vi "AsyncEngine.CAN.vi"(10 "Parameters":variant, 11 "Process":refnum<class "Process.lvclass">) -> ()   [LabVIEW 2015, in "Protection and Rolling Counter Addon Engine.lvlib"]
uses:
  Protection and Rolling Counter Addon Engine.lvlib
  <vilib>/NI/NIVS Inline Async API/_VS Inline Async API/Process/Process.lvclass
  Types/RT Async Engine Variables.ctl
  Types/RT Frame Settings.ctl
  Types/RT Protection Configuration.ctl
  Shared/Types/Protection Type.ctl
  Shared/Types/InputChannelConfiguration.ctl
  Types/RT Counter Settings.ctl
  Types/RT Data References.ctl
  <vilib>/NI/NIVS Inline Async API/_Data Access Engine/Data Access Engine/Types/Write.DVR.ctl
  <vilib>/NI/NIVS Inline Async API/_Data Access Engine/Access Type Classes/Write/Write.lvclass
  <vilib>/NI/NIVS Inline Async API/_Data Access Engine/Data Access Engine/Types/Read.DVR.ctl
  <vilib>/NI/NIVS Inline Async API/_Data Access Engine/Access Type Classes/Read/Read.lvclass
  <vilib>/NI/NIVS Inline Async API/_VS Inline Async API/Process/Process.lvclass/Process.ctl
  <vilib>/Platform/TimedLoop/XDataNode/timing_clust.ctl
  <vilib>/Platform/TimedLoop/XDataNode/nitl_modes.ctl
  <vilib>/Platform/TimedLoop/XDataNode/wakeup.ctl
  <vilib>/NI/NIVS Inline Async API/_VS Inline Async API/Process/Data Member Access/Read Data Access.vi
  <vilib>/NI/NIVS Inline Async API/_VS Inline Async API/Error Handling Process/SubVIs/Error.ConvertArray.vi
  <vilib>/NI/NIVS Inline Async API/_Data Access Engine/Data Access Engine/Methods/Write.Lookup.vi
  <vilib>/NI/NIVS Inline Async API/_Data Access Engine/Data Access Engine/Methods/Read.Lookup.vi
  Shared/SubVIs/GUID Lookup.vi
  <vilib>/platform/TimedLoop/XDataNode/XDataNode.xnode
  <vilib>/NI/NIVS Inline Async API/_Data Access Engine/Data Access Engine/Data Access Engine.lvclass
  Shared/Protection and Rolling Counter Addon Shared.lvlib
  <vilib>/Platform/TimedLoop/XDataNode/XDNodeRunTimeDep.lvlib
  <vilib>/NI Veristand/Custom Device Tools/Custom Device Utility Library/Custom Device Utility Library.lvlib
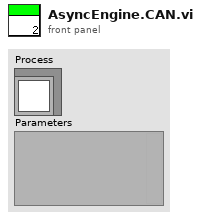
[diagram p1: front panel]
types:
  T1 = typedef "Protection and Rolling Counter Addon Engine.lvlib/RT Data References.ctl" = cluster{"ProtectionsAndCounters.Ref":T2, "Signals.Ref":T3, "Status.Ref":T2}
  T2 = typedef "Data Access Engine.lvlib/Data Access Engine.lvclass/Write.DVR.ctl" = refnum<data-value>
  T3 = typedef "Data Access Engine.lvlib/Data Access Engine.lvclass/Read.DVR.ctl" = refnum<data-value>
  T4 = typedef "Protection and Rolling Counter Addon Engine.lvlib/RT Async Engine Variables.ctl" = cluster{"CAN Session":refnum<k21>, "Frames":T5[], "Frame Count":i32}
  T5 = typedef "Protection and Rolling Counter Addon Engine.lvlib/RT Frame Settings.ctl" = cluster{"Frame ID":u32, "VS Offset":i32, "VS Length":i32, "Frame Conversion":refnum<k21>, "Generation Period":u32, "Time Since Last Generation":u32, "Has Protection?":bool, "Protection Configurations":T6[], "Has Counter":bool, "Counter Configurations":T9[], "Has Disable?":bool, "Disable VS Index":i32, "Frame.PrevData":dbl[], "Generation Iterations":u32, "Generation Counter":u32}
  T6 = typedef "Protection and Rolling Counter Addon Engine.lvlib/RT Protection Configuration.ctl" = cluster{"Protection Frame Index":i32, "Protection Type":T7, "Data Indeces":i32[], "Initialized Data Array":dbl[], "Check Sum Conversion":refnum<k21>, "CRC Channels":T8[], "Protection VS Index":i32}
  T7 = typedef "Protection and Rolling Counter Addon Shared.lvlib/Protection Type.ctl" = enum16{"Checksum", "CRC"}
  T8 = typedef "Protection and Rolling Counter Addon Shared.lvlib/InputChannelConfiguration.ctl" = cluster{"Start Bit":i32, "Name":string, "Number of bits":i32, "Scale":dbl, "Offset":dbl, "Data Type":u32}
  T9 = typedef "Protection and Rolling Counter Addon Engine.lvlib/RT Counter Settings.ctl" = cluster{"Counter Frame Index":i32, "Max Count":dbl, "Counter VS Index":i32}
  T10 = typedef "XDNodeRunTimeDep.lvlib/timing_clust.ctl" = cluster{"Expected End [f-1]":u64, "Actual End [f-1]":u64, "Finished Late? [f-1]":bool, "Expected End [i-1]":u64, "Actual End [i-1]":u64, "Finished Late? [i-1]":bool, "Expected Start [i]":u64, "Actual Start [i]":u64, "Expected Start [f]":u64, "Actual Start [f]":u64, "Source Name":string, "Structure Name":string, "Period":i64, "Deadline":i64, "Offset":i64, "Start":i64, "Priority":i32, "Timeout":i32, "Mode":T11, "Wakeup Reason":T12, "Error":errorcluster, "Source Type":string, "Secondary Source Type":string, "Global End Time":u64, "Global Start Time":u64, "Frame Duration":u64, "Iteration Duration":u64, "Assigned CPU":i32, "I/O Scan Engine Mode":u32}
  T11 = typedef "XDNodeRunTimeDep.lvlib/nitl_modes.ctl" = enum32{"No Change", "Process missed periods, maintain original phase", "Discard missed periods, maintain original phase", "Process missed periods, ignore original phase", "Discard missed periods, ignore original phase"}
  T12 = typedef "XDNodeRunTimeDep.lvlib/wakeup.ctl" = enum32{"Normal", "Aborted", "Asynchronous wakeup", "Timing source error", "Timed loop error", "Timeout"}
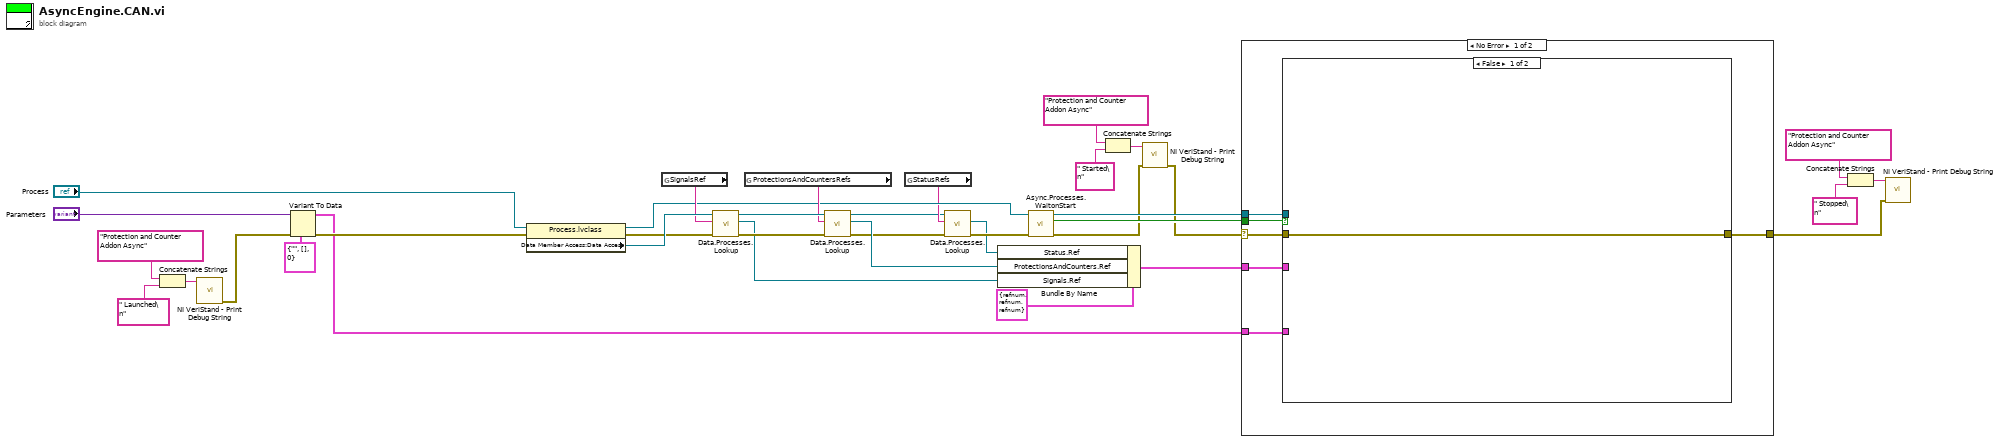
[diagram p0: block diagram]
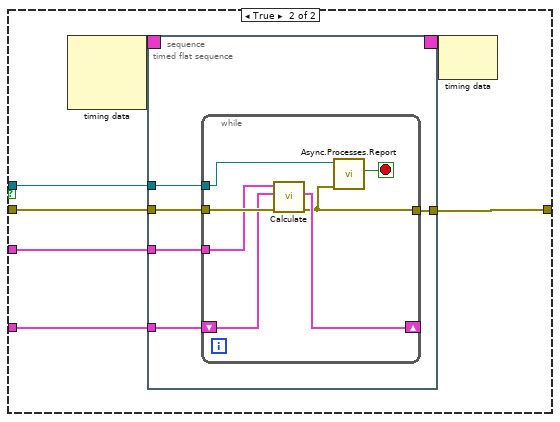
[diagram p2: hidden frame]
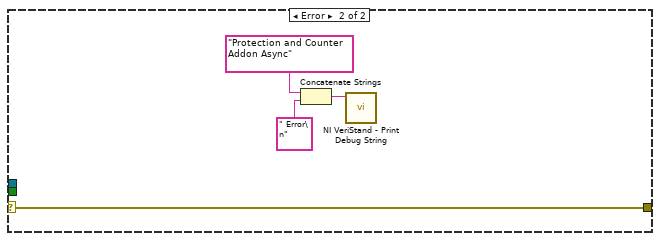
[diagram p3: hidden frame]
diagram:
  n1 = Concatenate Strings("Protection and Counter Addon Async" ("Debug String"), " Launched\n" ("string")) -> (w12:string)
  n2 = call <vilib>:"NI VeriStand - Print Debug String.vi"("Message"=w12) -> ("error out"=w10:errorcluster)  [unwired: 10 in]
  n3 = Variant To Data(error in=w10, type=T4 {"CAN Session"="", "Frames"=[], "Frame Count"=0} ("RT Configuration"), Variant="Parameters") -> (data=w20:T4, error out=w34:errorcluster)
  n4 = property class="Process.lvclass"(reference="Process", error in=w34) -> (reference out=w26:refnum<class "Process.lvclass">, error out=w30:errorcluster, "Data Member Access:Data Access"=w32:refnum<class "Data Access Engine.lvclass">)
  n5 = global read "GUID Lookup.vi" "SignalsRef"() -> (w28:string)
  n6 = call-poly <vilib>:"Data.Processes.Lookup.vi"("error in (no error)"=w30, "Name"=w28, "Data Access API in"=w32) -> ("error out"=w29:errorcluster, "Ref"=w24:T3, "Data Access API out"=w31:refnum<class "Data Access Engine.lvclass">)  [unwired: 5 in, 1 out]
  n7 = global read "GUID Lookup.vi" "ProtectionsAndCountersRefs"() -> (w27:string)
  n8 = call-poly <vilib>:"Data.Processes.Lookup.vi"("error in (no error)"=w29, "Name"=w27, "Data Access API in"=w31) -> ("error out"=w16:errorcluster, "Ref"=w23:T2, "Data Access API out"=w17:refnum<class "Data Access Engine.lvclass">)  [unwired: 5 in, 1 out]
  n9 = global read "GUID Lookup.vi" "StatusRefs"() -> (w18:string)
  n10 = call-poly <vilib>:"Data.Processes.Lookup.vi"("error in (no error)"=w16, "Name"=w18, "Data Access API in"=w17) -> ("error out"=w15:errorcluster, "Ref"=w14:T2)  [unwired: 5 in, 2 out]
  n11 = Bundle By Name(cluster=T1 {"ProtectionsAndCounters.Ref"=refnum, "Signals.Ref"=refnum, "Status.Ref"=refnum}, "Status.Ref"=w14, "ProtectionsAndCounters.Ref"=w23, "Signals.Ref"=w24) -> (w19:T1)
  n12 = call <vilib>:"Async.Processes.WaitonStart.vi"("error in (no error)"=w15, "Process"=w26) -> ("error out"=w6:errorcluster, "Execute"=w21:bool, "Process out"=w25:refnum<class "Process.lvclass">)  [unwired: 7 in]
  n13 = Concatenate Strings("Protection and Counter Addon Async" ("Debug String"), " Started\n" ("string")) -> (w8:string)
  n14 = call <vilib>:"NI VeriStand - Print Debug String.vi"("error in (no error)"=w6, "Message"=w8) -> ("error out"=w5:errorcluster)  [unwired: 9 in]
  n15 = case shown="No Error" w5 {
    selector: w5 -> [w38 w75]
    tunnel: w25 -> [w42 _]
    tunnel: w21 -> [w41 _]
    tunnel: w20 -> [w40 _]
    tunnel: w19 -> [w39 _]
    tunnel: [w37 w75] -> w1
    frame No Error {
      n16 = case shown="False" w41 {
        tunnel: w42 -> [_ w50]
        tunnel: w40 -> [_ w47]
        tunnel: w39 -> [_ w49]
        tunnel: w38 -> [w43 w48]
        tunnel: [w43 w44] -> w37
        frame False {
        }
        frame True {
          n17 = node-c288() -> (w46:T10)  [unwired: 3 in]
          n18 = timed-sequence {
            timing: w46 -> [_]
            timing-out: [_] -> w45
            tunnel: w50 -> [w55]
            tunnel: w47 -> [w54]
            tunnel: w49 -> [w53]
            tunnel: w48 -> [w52]
            tunnel: [w51] -> w44
            n19 = timed-flat-sequence {
              tunnel: w55 -> [w60]
              tunnel: w54 -> [w57]
              tunnel: w53 -> [w59]
              tunnel: w52 -> [w58]
              tunnel: [w56] -> w51
              n20 = while {
                tunnel: w60 -> [w67]
                tunnel: w59 -> [w62]
                tunnel: w58 -> [w66]
                shift-right: [w63] -> _
                shift-left: w57 -> [w65]
                tunnel: [w61] -> w56
                stop <- w64 stop-if-true
                n21 = call "Calculate.vi"("error in (no error)"=w66, "Async Settings"=w65, "Data Refs"=w62) -> ("error out"=w61:errorcluster, "Async Settings"=w63:T4)  [unwired: 7 in]
                n22 = call <vilib>:"Async.Processes.Report.vi"("Error"=w61, "Process in"=w67) -> ("Stop"=w64:bool)  [unwired: 8 in, 1 out]
              }
            }
          }
          n23 = node-c288(w45) -> ()  [unwired: 1 out]
        }
      }
    }
    frame Error {
      n24 = Concatenate Strings("Protection and Counter Addon Async" ("Debug String"), " Error\n" ("string")) -> (w73:string)
      n25 = call <vilib>:"NI VeriStand - Print Debug String.vi"("Message"=w73) -> ()  [unwired: 10 in, 1 out]
    }
  }
  n26 = Concatenate Strings("Protection and Counter Addon Async" ("Debug String"), " Stopped\n" ("string")) -> (w3:string)
  n27 = call <vilib>:"NI VeriStand - Print Debug String.vi"("error in (no error)"=w1, "Message"=w3) -> ()  [unwired: 9 in, 1 out]
